vi "rad_FTP Put File Wrapper.vi"(4 "active (F)":bool, 5 "password":string, 6 "binary (T)":bool=TRUE, 7 "user (admin)":string="admin", 8 "error in (no error)":errorcluster, 9 "local path":path, 10 "remote path":string, 11 "Target settings":T1={"Hostname"="", "Serial number"="", "Product name"="", "Product code"=0, "System status"="", "Credential type"=enum."None/Unlocked", "User added?"=FALSE, "Primary NIC"={"MAC address"="", "IP Address Request Mode"=2, "IP address"="", "Subnet mask"="", "Gateway"="", "DNS server"=""}} {"Primary NIC"."IP Address Request Mode" items=["Static"=1, "DHCP/Link-Local"=2, "Link-Local Only"=4, "DHCP Only"=8]}) -> (0 "error out":errorcluster)   [LabVIEW 2020]
uses:
  <vilib>/nisyscfg/nisyscfg.lvlib
  <vilib>/nisyscfg/Close (System).vi
  <vilib>/FTP/NI_FTP.lvlib
  Targets/TypeDefs/rad_Target Information.ctl
  Targets/TypeDefs/rad_Target Network Settings.ctl
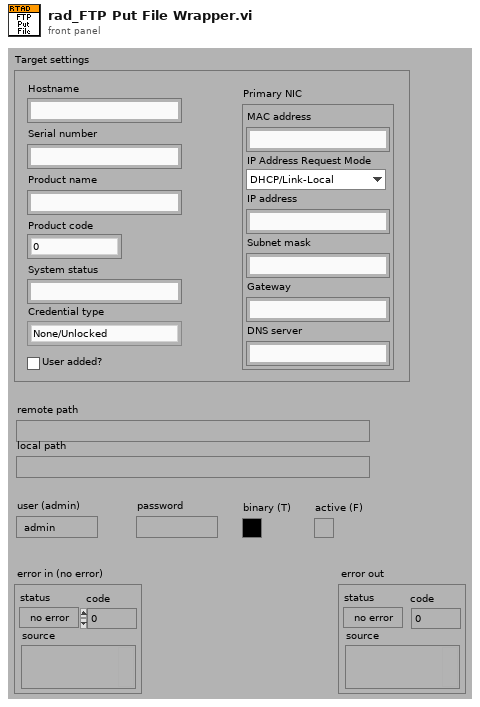
[diagram p1: front panel]
types:
  T1 = typedef "rad_Target Information.ctl" = cluster{"Hostname":string, "Serial number":string, "Product name":string, "Product code":i32, "System status":string, "Credential type":enum16{"None/Unlocked", "FTP Password", "NIAuth Credentials"}, "User added?":bool, "Primary NIC":T2}
  T2 = typedef "rad_Target Network Settings.ctl" = cluster{"MAC address":string, "IP Address Request Mode":i32, "IP address":string, "Subnet mask":string, "Gateway":string, "DNS server":string}
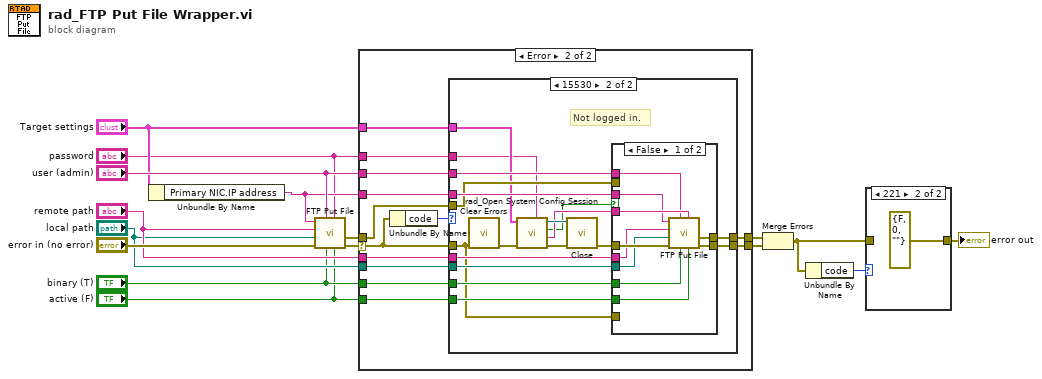
[diagram p0: block diagram]
diagram:
  n1 = Unbundle By Name("Target settings") -> ("Primary NIC.IP address"=w3:string)
  n2 = call <vilib>:"FTP Put File.vi"("active (T)"="active (F)", "password"="password", "binary (F)"="binary (T)", "user"="user (admin)", "error in (no error)"="error in (no error)", "local path"="local path", "remote path"="remote path", "host"=w3) -> ("error out"=w12:errorcluster, "file error"=w10:errorcluster)  [unwired: 2 in]
  n3 = case shown="Error" w12 {
    selector: w12 -> [w18 w25]
    tunnel: [w18 w31] -> w11
    tunnel: w3 -> [_ w30]
    tunnel: "remote path" -> [_ w29]
    tunnel: "local path" -> [_ w28]
    tunnel: "binary (T)" -> [_ w27]
    tunnel: "active (F)" -> [_ w26]
    tunnel: w10 -> [w17 w23]
    tunnel: [w17 w22] -> w5
    tunnel: "user (admin)" -> [_ w21]
    tunnel: "Target settings" -> [_ w20]
    tunnel: "password" -> [_ w19]
    frame No Error {
    }
    frame Error {
      n4 = Unbundle By Name(w25) -> ("code"=w24:i32)
      n5 = case shown="15530" w24 {
        tunnel: w25 -> [w33 w39]
        tunnel: [w33 w47] -> w31
        tunnel: w30 -> [_ w45]
        tunnel: w29 -> [_ w44]
        tunnel: w28 -> [_ w43]
        tunnel: w27 -> [_ w42]
        tunnel: w26 -> [_ w41]
        tunnel: w23 -> [w32 w38]
        tunnel: [w32 w37] -> w22
        tunnel: w21 -> [_ w36]
        tunnel: w20 -> [_ w35]
        tunnel: w19 -> [_ w34]
        frame Default {
        }
        frame 15530 {
          # "Not logged in."
          n6 = call <vilib>:"Clear Errors.vi"("error in (no error)"=w39) -> ("error out"=w49:errorcluster)  [unwired: 5 in, 1 out]
          n7 = call "rad_Open System Config Session.vi"("Password"=w34, "error in (no error)"=w49, "Target settings"=w35) -> ("error out"=w50:errorcluster, "Password out"=w46:string, "Cancelled"=w40:bool, "Session out"=w51:refnum<k21>)  [unwired: 5 in]
          n8 = call-poly <vilib>:"Close.vi"("error in (no error)"=w50, "Session in"=w51) -> ("error out"=w48:errorcluster)  [unwired: 9 in]
          n9 = case shown="False" w40 {
            tunnel: w48 -> [w60 _]
            tunnel: [w61 w63] -> w47
            tunnel: w46 -> [w58 _]
            tunnel: w45 -> [w56 _]
            tunnel: w44 -> [w57 _]
            tunnel: w43 -> [w55 _]
            tunnel: w42 -> [w54 _]
            tunnel: w41 -> [w53 _]
            tunnel: w39 -> [_ w63]
            tunnel: [w59 w62] -> w37
            tunnel: w38 -> [_ w62]
            tunnel: w36 -> [w52 _]
            frame False {
              n10 = call <vilib>:"FTP Put File.vi"("active (T)"=w53, "password"=w58, "binary (F)"=w54, "user"=w52, "error in (no error)"=w60, "local path"=w55, "remote path"=w57, "host"=w56) -> ("error out"=w61:errorcluster, "file error"=w59:errorcluster)  [unwired: 2 in]
            }
            frame True {
            }
          }
        }
      }
    }
  }
  n11 = Merge Errors(w5, w11) -> (w13:errorcluster)
  n12 = Unbundle By Name(w13) -> ("code"=w14:i32)
  n13 = case shown="221" w14 {
    tunnel: w13 -> [w64 _]
    tunnel: [w64 errorcluster {"status"=FALSE, "code"=0, "source"=""} ("error IO")] -> w15
    frame Default {
    }
    frame 221 {
    }
  }
  "error out" <- w15
